vi "Dashboard Main.vi"() -> ()   [LabVIEW 2023]
uses:
  Support/Utility/FP_Size VI to Decoration Simple.vi/TypeDefs_Utility/Cluster_FP Set.ctl
  Support/Utility/FP_Size VI to Decoration Simple.vi/TypeDefs_Utility/ENUM RB_Pos_Quadrant Position.ctl
  <vilib>/event_ctls.llb/eventvkey.ctl
  <vilib>/Rock Robotics/Network Tables/NT Read Numeric Array.vi
  <vilib>/Rock Robotics/WPI/Dashboard/WPI_DashboardLogging Global.vi
panel:
  in  "Camera Settings Right":T1={"Frame Rate"=30, "Compression"=30, "Size"=1, "DB Camera Config"=FALSE} {"Frame Rate" scale=1.0..30.0; "Compression" scale=100.0..-1.0; "Size" items=["640x480", "320x240", "160x120"]}
  in  "Camera Name Right":string(combo)="No Camera Selection"
  out "Camera Perf":string
  in  "Camera Settings":T1={"Frame Rate"=30, "Compression"=30, "Size"=1, "DB Camera Config"=FALSE} {"Frame Rate" scale=1.0..30.0; "Compression" scale=100.0..-1.0; "Size" items=["640x480", "320x240", "160x120"]}
  in  "TCP":refnum<k5>
  in  "Rec Mode":enum32{"Stop", "Record", "Playback"}(radio)
  out "Robot IP":string
  out "Image Message":string="Timeout in Camera Communications"
  in  "Dashboard Tab":T2(tab)
  in  "Select Auto":string(combo)="Select Autonomous ..."
  out "NT Connection":bool
  out "MotorChart R":cluster{"Numeric":dbl, "Numeric":dbl}(graph)
  out "MotorChart L":cluster{"Numeric":dbl, "Numeric":dbl}(graph)
  out "MotorSliders R":cluster{"MotorSlide1":dbl, "MotorSlide2":dbl} {"MotorSlide2" scale=-1.0..1.0 scale format="%#_2e"; "MotorSlide1" scale=-1.0..1.0 scale format="%#_2e"}
  out "MotorSliders L":cluster{"MotorSlide1":dbl, "MotorSlide2":dbl} {"MotorSlide2" scale=-1.0..1.0 scale format="%#_2e"; "MotorSlide1" scale=-1.0..1.0 scale format="%#_2e"}
  out "Gyro":dbl(knob) scale=0.0..360.0
  out "JS1 Z":dbl(slide) scale=-1.0..1.0 scale format="%#_2e"
  out "JS1 Graph":cluster{"X":dbl, "Y":dbl}[](graph)
  out "JS1 Buttons":T3
  out "JS2 Z":dbl(slide) scale=-1.0..1.0 scale format="%#_2e"
  out "JS2 Graph":cluster{"X":dbl, "Y":dbl}[](graph)
  out "JS2 Buttons":T3
  out "Mode":T4(ring)=enum."Auto Disabled"
  out "Right Camera Perf":cluster{"Bandwidth (Mbps)":dbl, "FPS":dbl}
  out "Camera Image Right":T5(plugin-control)
  in  "DB/String 9":string
  in  "DB/String 8":string
  in  "DB/String 7":string
  in  "DB/String 6":string
  in  "DB/String 5":string
  in  "DB/String 4":string
  in  "DB/String 3":string
  in  "DB/String 2":string
  in  "DB/String 1":string
  in  "DB/String 0":string
  in  "DB/Slider 0":dbl(slide) scale=0.0..5.0
  in  "DB/Slider 1":dbl(slide) scale=0.0..5.0
  in  "DB/Slider 2":dbl(slide) scale=0.0..5.0
  in  "DB/Slider 3":dbl(slide) scale=0.0..5.0
  out "DB/LED 3":bool
  out "DB/LED 2":bool
  out "DB/LED 1":bool
  out "DB/LED 0":bool
  in  "DB/Button 3":bool
  in  "DB/Button 2":bool
  in  "DB/Button 1":bool
  in  "DB/Button 0":bool caption="New Name"
  in  "Test Slider":dbl(slide) scale=0.0..100.0 scale format="%#_3g"
  in  "On/Off":bool caption="Solenoid"
  in  "Test Name":u16(ring) items=["Select the test to run..."]
  in  "Test Tree":string(tree)
  in  "Motor":cluster{"Value":dbl, "Enable":bool} {"Value" scale=-1.0..1.0 scale format="%#_3g"}
  out "Progress":T6 {"Test Progress" scale=0.0..100.0}
  in  "Rev/Fwd":cluster{"Forward":bool, "Reverse":bool}
  in  "Test Ring":u16(ring) items=["Monochrome", "Color"]
  in  "CheckList":i32(listbox)
  out "Tree":string(tree)
  out "Camera Image":T5(plugin-control)
  out "Background":bool
  in  "Camera Name":string(combo)="No Camera Selection"
  # "HW"
  # "HW"
  # "Joysticks"
  # "Drive Motors"
  # "Front"
  # "Right"
  # "Left"
  # "Back"
  # "This tab is a great place for autonomous settings and robot-specific values.\nPlace controls and indicators inside this tab and match name to\nDashboard Variables on robot. You can also delete this comment."
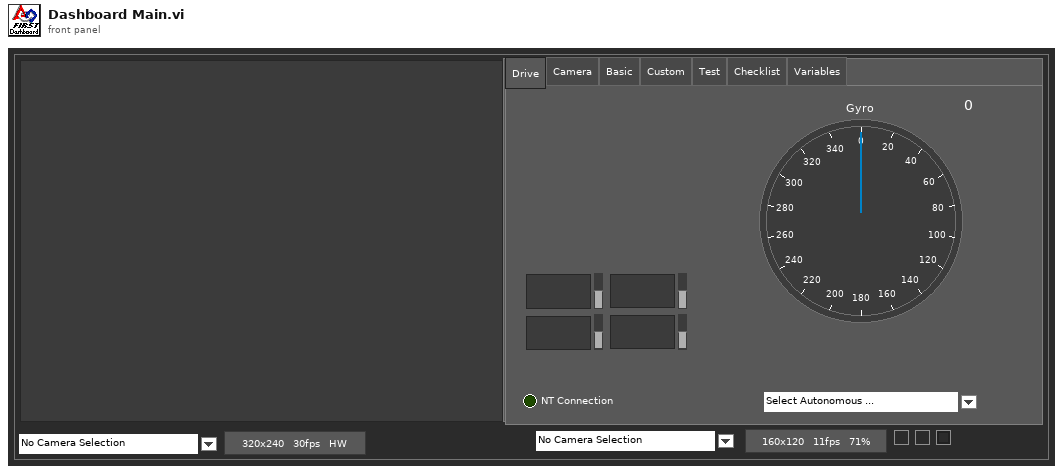
[diagram p1: front panel]
types:
  T1 = cluster{"Frame Rate":i32, "Compression":i32, "Size":u16, "DB Camera Config":bool}
  T2 = enum32{"Drive", "Camera", "Basic", "Custom", "Test", "Checklist", "Variables"}
  T3 = cluster{bool, bool, bool, bool, bool, bool, bool, bool, bool, bool, bool, bool}
  T4 = enum8{"Tele-Op Disabled", "Tele-Op Enabled", "Auto Disabled", "Auto Enabled", "Test Disabled", "Test Enabled", "Disconnected", "No Code", "E-Stop"}
  T5 = typedef "IMAQ Image.ctl" = refnum<image>
  T6 = cluster{"Test Progress":u8, "Test Progress Text":string}
  T7 = typedef "Cluster_FP Set.ctl" = cluster{"Menu Bar":bool, "Position":T8, "Decoration index":i32, "border(px)":i32, "Monitor #":i32}
  T8 = typedef "ENUM RB_Pos_Quadrant Position.ctl" = enum32{"LFT-TOP", "MID-TOP", "RGT-TOP", "LFT-CTR", "MID-CTR", "RGT-CTR", "LFT-BOT", "MID-BOT", "RGT-BOT"}
  T9 = cluster{"Save Path":path, "Interval (s)":dbl, "Keep":i32}
  T10 = enum32{"Drive", "Camera", "Basic", "Custom", "Test", "Commands", "Checklist", "Variables"}
  T11 = typedef "Image Type" = u32
  T12 = cluster{"Error Strings":string, "Disable Counts":cluster{u16, u16}, "Rail Faults":cluster{u16, u16, u16}, "Robot IP":string, "DB Mode":u8, "Event Info":cluster{"Name":string, "Type":u8, "Number":u16, "Replay":u8}}
  T13 = cluster{"Storage":cluster{"Disk Free":u64, "RAM Block":u32, "RAM free":u32}, "CPU Utilization":cluster{"CPU % ISR":sgl, "CPU % Time Crit":sgl, "CPU % Timed Str":sgl, "CPU % High":sgl, "CPU % Above":sgl, "CPU % Normal":sgl, "CPU % Low":sgl}, "CAN":cluster{"% Bus Utilization":sgl, "Bus Off Cnt":u32, "TX_FIFO Full Cnt":u32, "Receive Error Cnt":u8, "Transmit Error Cnt":u8}, "HID":cluster{"HID Outputs":u32, "Rumble Low":u16, "Rumble High":u16}[]}
  T14 = cluster{"Status bits":cluster{"Test Mode":bool, "Autonomous":bool, "Enabled":bool, "Code Start":bool, "Brownout":bool, "Reserved 2":bool, "Reserved 3":bool, "E-Stop":bool}, "Code Trace":cluster{"Disabled":bool, "TeleOp":bool, "Auto":bool, "Test":bool}, "Controller Type":enum16{"unknown", "cRIO", "roboRio"}, "Code?":enum16{"unknown", "noCode", "code"}, "Battery V":dbl}
  T15 = cluster{"Control Bits":cluster{"TestMode":bool, "Autonomous":bool, "Enabled":bool, "FMS Present":bool, bool, bool, bool, "E-Stop":bool}, "Team Station ":u8, "Countdown":sgl, "Joystick Values":cluster{"Axes":dbl[], "Buttons":bool[], "POVs":i16[]}[]}
  T16 = cluster{"Axes":dbl[], "Buttons":bool[], "POVs":i16[]}[]
  T17 = cluster{"Axes":dbl[], "Buttons":bool[], "POVs":i16[]}
  T18 = cluster{"Buttons[0]":bool, "Buttons[1]":bool, "Buttons[2]":bool, "Buttons[3]":bool, "Buttons[4]":bool, "Buttons[5]":bool, "Buttons[6]":bool, "Buttons[7]":bool, "Buttons[8]":bool, "Buttons[9]":bool, "Buttons[10]":bool, "Buttons[11]":bool}
  T19 = cluster{"Global Rectangle":i32[], "Contours":cluster{"Contour Type":u32, "ROI Type":u32, "Points":i32[]}[]}
  T20 = cluster{"Camera Name":string, string, "Saved DB Images Info":cluster{"Save Path":path, "Interval (s)":dbl, "Keep":i32}}
  T21 = cluster{"Camera Name Right":string, string, "Saved DB Images Info":cluster{"Save Path":path, "Interval (s)":dbl, "Keep":i32}}
  T22 = cluster{"Operation":enum16{"Update", "Clear"}, "Color Box":u32}[]
  T23 = typedef "eventvkey.ctl" = enum16{"ASCII", "Enter", "Return", "Shift", "Ctrl", "Alt", "Cmd", "Opt", "Caps", "NumLock", "Clear", "Break", "Up", "Down", "Left", "Right", "Insert", "Delete", "Home", "End", "PageUp", "PageDown", "Escape", "Help", "Pause", "ScrollLock", "F1", "F2", "F3", "F4", "F5", "F6", "F7", "F8", "F9", "F10", "F11", "F12", "F13", "F14", "F15", "F16", "F17", "F18", "F19", "F20", "F21", "F22", "F23", "F24", "Play", "VolumeUp", "VolumeDown", "Mute", "Two Byte Char"}
  T24 = cluster{"Image Size":bool, "Image Type":bool, "Pixel Value":bool, "ROI Information":bool, "Zoom Factor":bool}
  T25 = cluster{"Operation":enum16{"Update", "Clear"}, "Color Box":u32}
  T26 = cluster{"Shift":bool, "Ctrl":bool, "Alt":bool, "Cmd":bool, "Opt":bool}
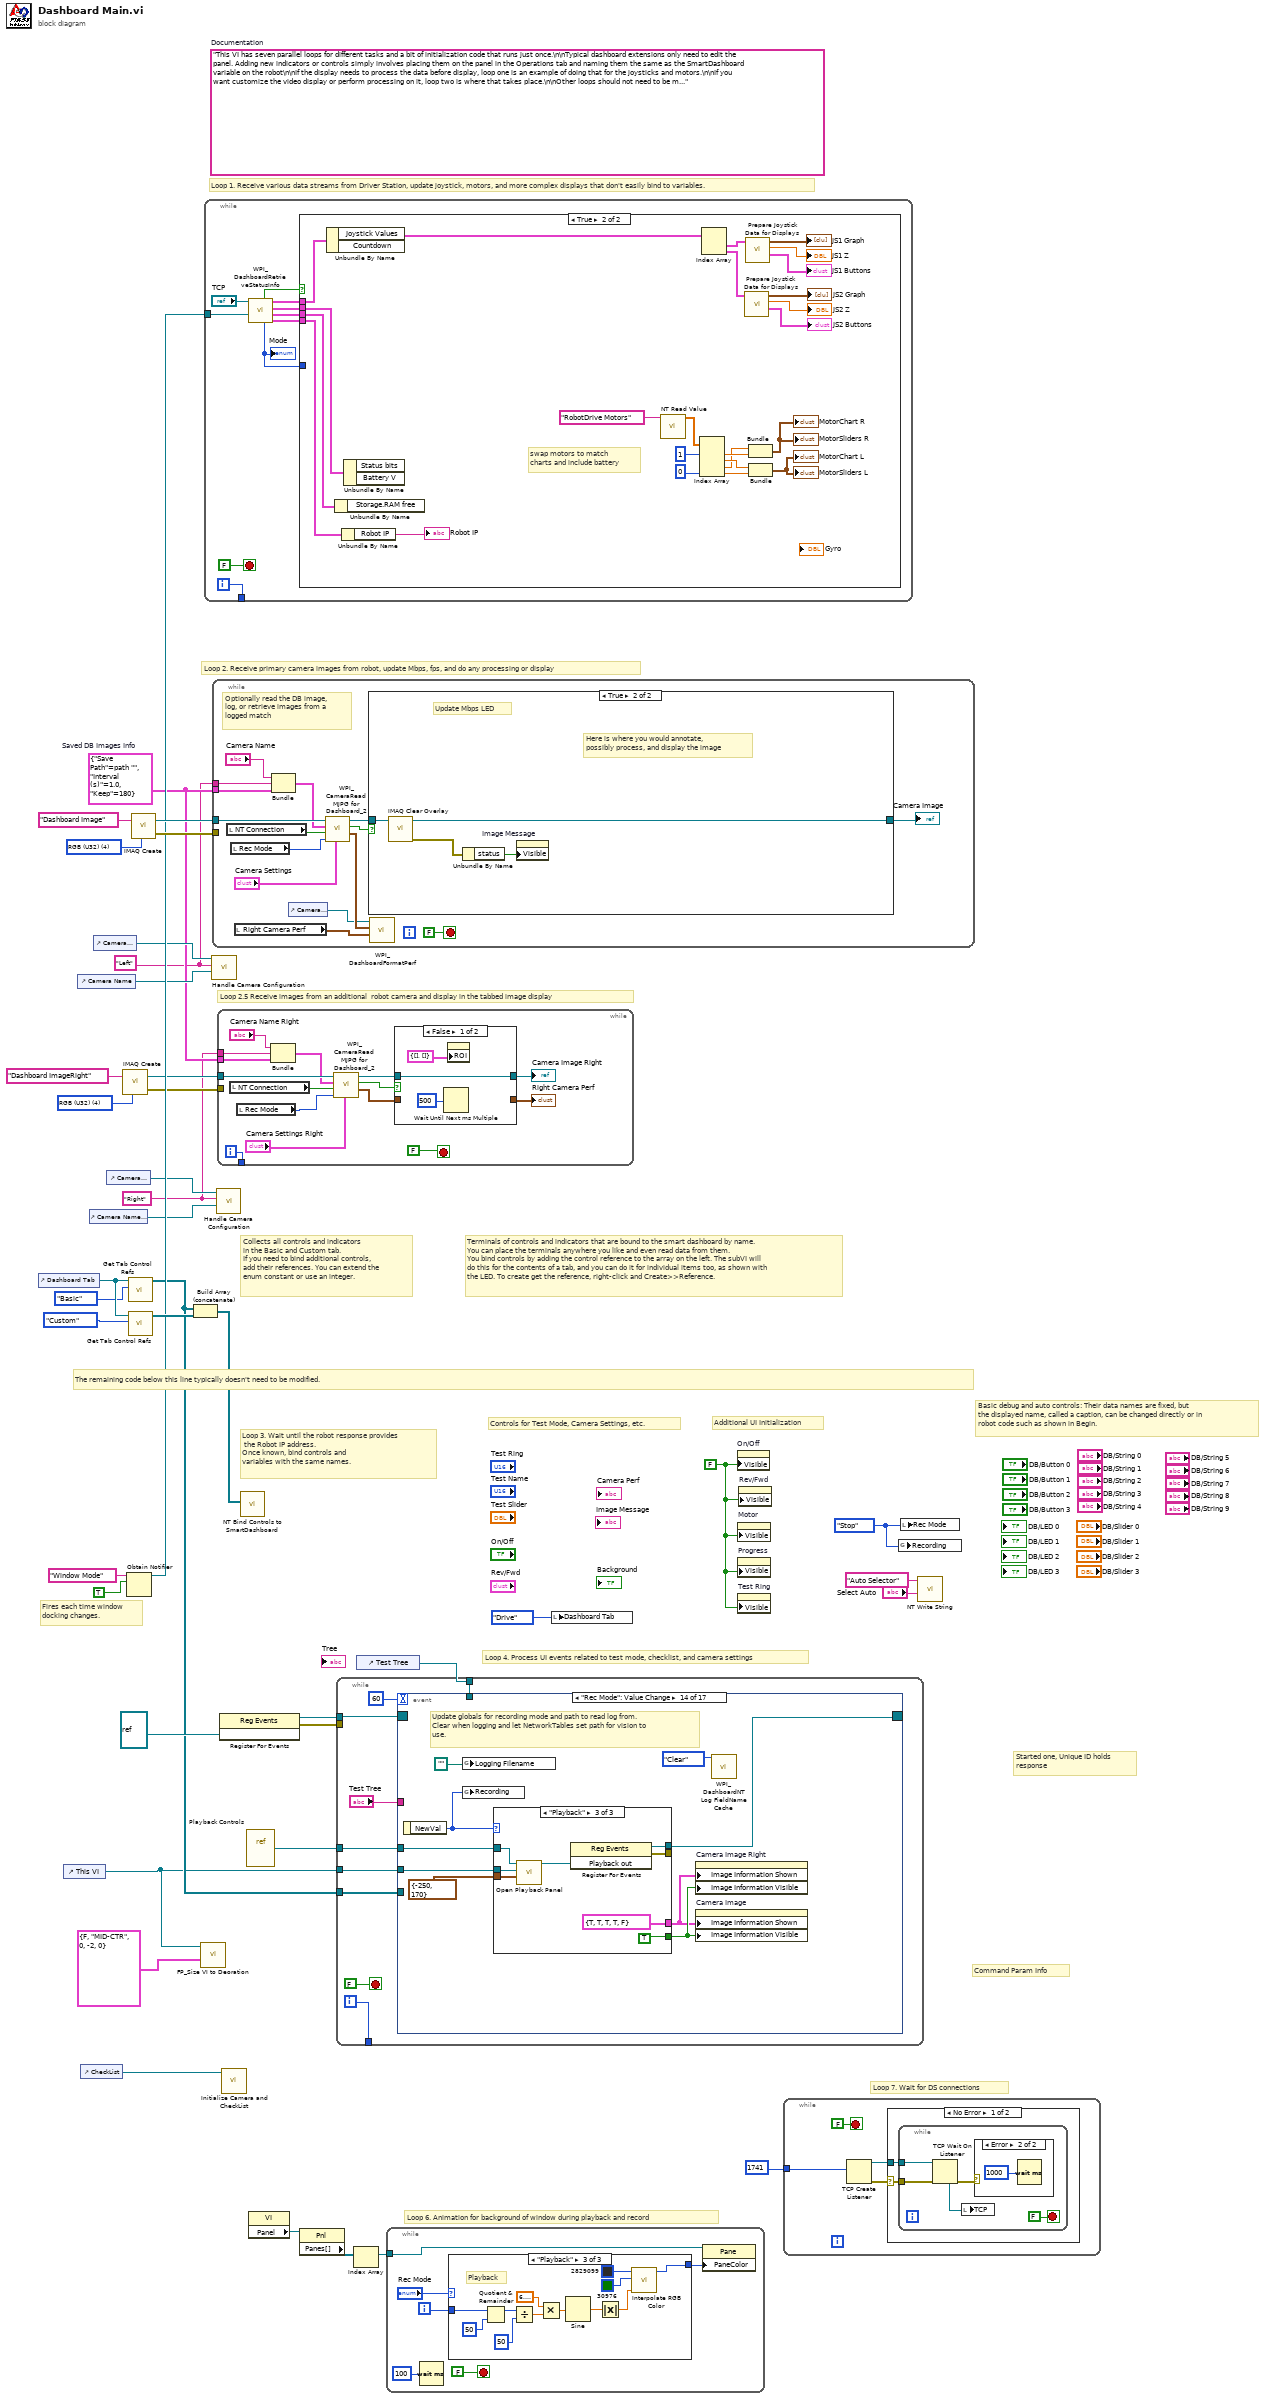
[diagram p0: block diagram]
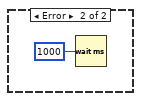
[diagram p4: hidden frame]
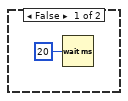
[diagram p5: hidden frame]
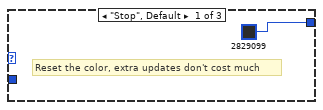
[diagram p6: hidden frame]
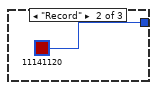
[diagram p7: hidden frame]
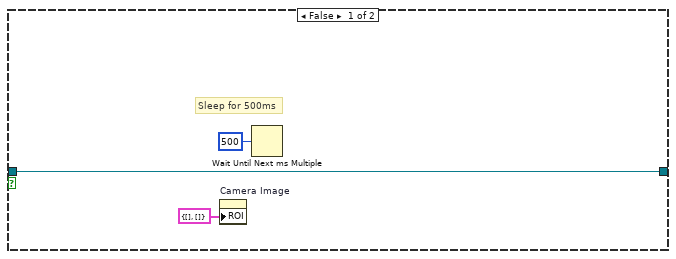
[diagram p8: hidden frame]
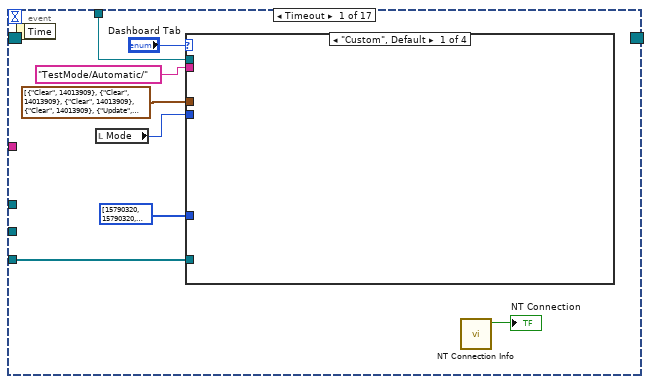
[diagram p9: hidden frame]
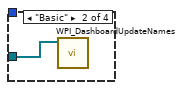
[diagram p10: hidden frame]
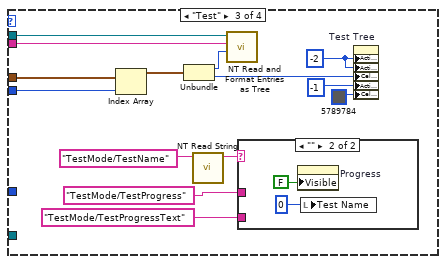
[diagram p11: hidden frame]
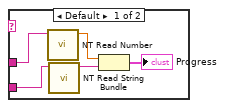
[diagram p12: hidden frame]
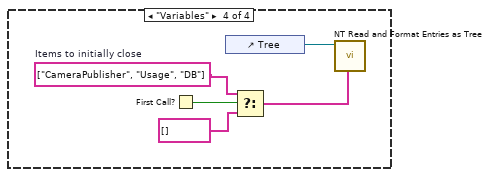
[diagram p13: hidden frame]
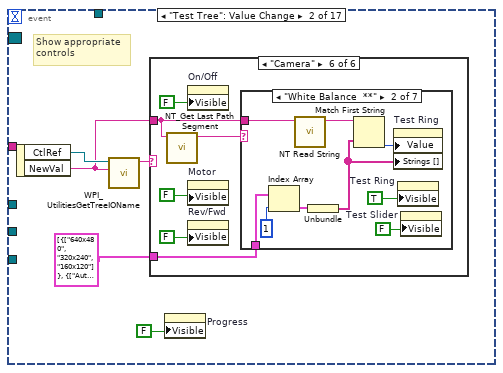
[diagram p14: hidden frame]
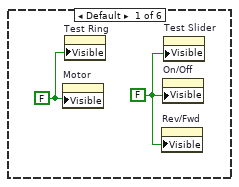
[diagram p15: hidden frame]
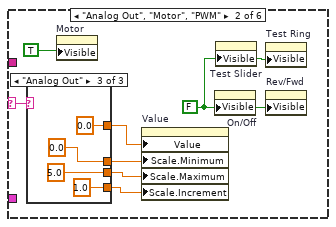
[diagram p16: hidden frame]
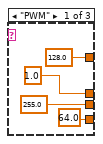
[diagram p17: hidden frame]
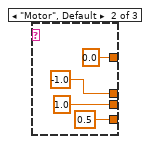
[diagram p18: hidden frame]
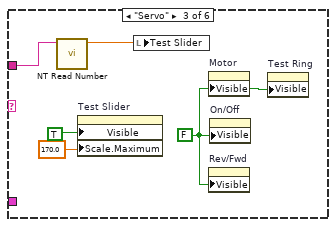
[diagram p19: hidden frame]
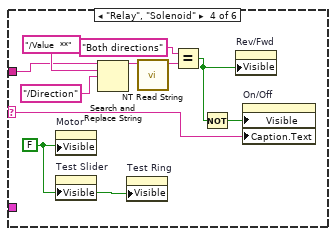
[diagram p20: hidden frame]
diagram:
  w5 = T9 {"Save Path"=path "", "Interval (s)"=1.0, "Keep"=180}  # Saved DB Images Info
  w4 = "Right"
  w3 = "Left"
  w12 = T11 4 items=["Grayscale (U8)", "Grayscale (I16)", "Grayscale (SGL)", "Complex (CSG)", "RGB (U32)", "HSL (U32)", "RGB (U64)"] ("Image Type")
  w27 = enum32{"Stop", "Record", "Playback"}."Stop" ("Rec Mode")
  w22 = FALSE ("Visible")
  (unwired) "This VI has seven parallel loops for different tasks and a bit of initialization code that runs just once.\n\nTypical dashboard extensions only need to edit the panel. Adding new indicators or controls simply involves placing them on the panel in the Operations tab and naming them the same as the SmartDashboard variable on the robot\n\nIf the display needs to process the data before display, loop one is an example of doing that for the joysticks and motors.\n\nIf you want customize the video display or perform processing on it, loop two is where that takes place.\n\nOther loops should not need to be modified. They are pretty standard, and document the task they perform."  # Documentation
  w41 = T11 4 items=["Grayscale (U8)", "Grayscale (I16)", "Grayscale (SGL)", "Complex (CSG)", "RGB (U32)", "HSL (U32)", "RGB (U64)"] ("Image Type")
  # "Loop 2.5 Receive images from an additional  robot camera and display in the tabbed image display"
  # "Command Param Info"
  # "Started one, Unique ID holds\nresponse"
  # "Loop 7. Wait for DS connections"
  # "Basic debug and auto controls: Their data names are fixed, but\nthe displayed name, called a caption, can be changed directly or in\nrobot code such as shown in Begin."
  # "Controls for Test Mode, Camera Settings, etc."
  # "Additional UI Initialization"
  # "Loop 6. Animation for background of window during playback and record"
  # "Fires each time window\ndocking changes."
  # "Collects all controls and indicators\nin the Basic and Custom tab.\nIf you need to bind additional controls,\nadd their references. You can extend the\nenum constant or use an integer."
  # "The remaining code below this line typically doesn't need to be modified."
  # "Loop 4. Process UI events related to test mode, checklist, and camera settings"
  # "Terminals of controls and indicators that are bound to the smart dashboard by name.\nYou can place the terminals anywhere you like and even read data from them.\nYou bind controls by adding the control reference to the array on the left. The subVI will\ndo this for the contents of a tab, and you can do it for individual items too, as shown with\nthe LED. To create get the reference, right-click and Create>>Reference."
  # "Loop 3. Wait until the robot response provides\n the Robot IP address.\nOnce known, bind controls and\nvariables with the same names."
  # "Loop 1. Receive various data streams from Driver Station, update joystick, motors, and more complex displays that don't easily bind to variables."
  # "Loop 2. Receive primary camera images from robot, update Mbps, fps, and do any processing or display"
  n1 = control-ref of="Dashboard Tab"() -> (w26:refnum<vi>)
  n2 = control-ref of="This VI"() -> (w2:refnum<vi>)
  n3 = control-ref of="Camera Name"() -> (w17:refnum<vi>)
  n4 = control-ref of="CheckList"() -> (w23:refnum<vi>)
  n5 = control-ref of="Camera Name Right"() -> (w8:refnum<vi>)
  n6 = control-ref of="Camera Settings"() -> (w18:refnum<vi>)
  n7 = control-ref of="Camera Settings Right"() -> (w9:refnum<vi>)
  n8 = call "IMAQ Create"("Image Name"="Dashboard ImageRight", "Image Type"=w12) -> ("New Image"=w11:T5, "error out"=w10:errorcluster)  [unwired: 2 in, 1 out]
  n9 = Obtain Notifier(name (unnamed)="Window Mode", notification data type=TRUE) -> (notifier out=w21:refnum<notifier>)  [unwired: 2 in, 2 out]
  n10 = call <vilib>:"Get Tab Control Refs.vi"("Page Index"=T10."Basic" ("Dashboard Tab"), "TabControl in"=w26) -> ("ControlsOnPage"=w16:refnum<vi>[])  [unwired: 9 in]
  n11 = call <vilib>:"Get Tab Control Refs.vi"("Page Index"=T10."Custom" ("Dashboard Tab"), "TabControl in"=w26) -> ("ControlsOnPage"=w25:refnum<vi>[])  [unwired: 9 in]
  n12 = call "IMAQ Create"("Image Name"="Dashboard Image", "Image Type"=w41) -> ("New Image"=w39:T5, "error out"=w38:errorcluster)  [unwired: 2 in, 1 out]
  n13 = Build Array (concatenate)(w16, w25) -> (w24:refnum<vi>[])
  n14 = call "FP_Size VI to Deoration.vi"("FPSet"=T7 {"Menu Bar"=FALSE, "Position"=enum."MID-CTR", "Decoration index"=0, "border(px)"=-2, "Monitor #"=0}, "VI Ref"=w2) -> ()  [unwired: 8 in, 2 out]
  n15 = while {
    tunnel: [w50] -> _
    tunnel: w21 -> [w42]
    i -> [w50]
    stop <- FALSE stop-if-true
    n16 = call <vilib>:"WPI_DashboardRetrieveStatusInfo.vi"("Window Mode Notifier"=w42, "TCP Cnx"="TCP") -> ("Power and Errors"=w45:T12, "Robot Metrics"=w48:T13, "Status Info"=w49:T14, "Control Info"=w46:T15, "Robot Mode"=w44:T4, "Process?"=w47:bool)  [unwired: 4 in]
    "Mode" <- w44
    n17 = case shown="True" w47 {
      tunnel: w49 -> [_ w76]
      tunnel: w48 -> [_ w75]
      tunnel: w46 -> [_ w74]
      tunnel: w45 -> [_ w73]
      tunnel: w44 -> [_ _]
      frame False {
        n18 = Wait (ms)(milliseconds to wait=u32 20) -> ()  [unwired: 1 out]
      }
      frame True {
        # "swap motors to match\ncharts and include battery"
        n19 = Unbundle By Name(w74) -> ("Joystick Values"=w64:T16)  [unwired: 1 out]
        n20 = Unbundle By Name(w75) -> ()  [unwired: 1 out]
        n21 = Unbundle By Name(w73) -> ("Robot IP"=→"Robot IP":string)
        n22 = Unbundle By Name(w76) -> ()  [unwired: 2 out]
        n23 = call-poly <vilib>:"NT Read Value.vi"("name"="RobotDrive Motors" ("Name")) -> ("value"=w54:dbl[])  [unwired: 8 in, 2 out]
        n24 = Index Array(array=w54, index #1=1, index #4=0) -> (element #1=w68:dbl, element #2=w69:dbl, element #3=w67:dbl, element #4=w72:dbl)  [unwired: 2 in]
        n25 = Index Array(array=w64) -> (element #1=w63:T17, element #2=w59:T17)  [unwired: 2 in]
        n26 = call "Prepare Joystick Data for Displays.vi"("Joystick Values"=w59) -> ("Buttons"=→"JS2 Buttons":T18, "Z Axis"=→"JS2 Z":dbl, "Cartesian Data"=→"JS2 Graph":cluster{"X axis":dbl, "X axis":dbl}[])  [unwired: 8 in]
        n27 = call "Prepare Joystick Data for Displays.vi"("Joystick Values"=w63) -> ("Buttons"=→"JS1 Buttons":T18, "Z Axis"=→"JS1 Z":dbl, "Cartesian Data"=→"JS1 Graph":cluster{"X axis":dbl, "X axis":dbl}[])  [unwired: 8 in]
        n28 = Bundle("Numeric"=w67, "Numeric"=w68) -> (→"MotorChart R" →"MotorSliders R":cluster{"Numeric":dbl, "Numeric":dbl})  [unwired: 1 in]
        n29 = Bundle("Numeric"=w69, "Numeric"=w72) -> (→"MotorChart L" →"MotorSliders L":cluster{"Numeric":dbl, "Numeric":dbl})  [unwired: 1 in]
      }
    }
  }
  n30 = call "Handle Camera Configuration.vi"("CameraNameRef"=w17, "Display Name"=w3, "ClusterRef"=w18) -> ()  [unwired: 9 in]
  n31 = while {
    tunnel: w39 -> [w90]
    tunnel: w38 -> [_]
    tunnel: w5 -> [w83]
    tunnel: w3 -> [w80]
    stop <- FALSE stop-if-true
    # "Optionally read the DB image,\nlog, or retrieve images from a\nlogged match"
    n32 = local read "NT Connection"() -> (w84:bool)
    n33 = local read "Rec Mode"() -> (w87:enum32{"Stop", "Record", "Playback"})
    n34 = local read "Right Camera Perf"() -> (w78:cluster{"Bandwidth (Mbps)":dbl, "FPS":dbl})
    n35 = Bundle("Camera Name"="Camera Name", w80, "Saved DB Images Info"=w83) -> (w82:T20)  [unwired: 1 in]
    n36 = control-ref of="Camera Perf"() -> (w77:refnum<vi>)
    n37 = call <vilib>:"WPI_CameraRead MJPG for Dashboard_2.vi"("Camera Settings"="Camera Settings", "Rec Mode"=w87, "NT Connection"=w84, "Capture Info"=w82, "Image in"=w90) -> ("perf info"=w79:cluster{"Bandwidth (Mbps)":dbl, "fps":dbl}, "Active"=w88:bool, "Image\\ out"=w89:T5)  [unwired: 4 in]
    n38 = case shown="True" w88 {
      tunnel: w89 -> [w93 w96]
      tunnel: [w93 w95] -> w85
      frame False {
        # "Sleep for 500ms"
        n39 = property on="Camera Image" class="ImageControl"("ROI"=T19 {"Global Rectangle"=[], "Contours"=[]}) -> ()  [unwired: 2 in, 2 out]
        n40 = Wait Until Next ms Multiple(millisecond multiple=u32 500) -> ()  [unwired: 1 out]
      }
      frame True {
        # "Here is where you would annotate,\npossibly process, and display the image"
        # "Update Mbps LED"
        n41 = call "IMAQ Clear Overlay"("Image"=w96) -> ("error out"=w97:errorcluster, "Image Out"=w95:T5)  [unwired: 2 in, 7 out]
        n42 = Unbundle By Name(w97) -> ("status"=w98:bool)
        n43 = property on="Image Message" class="Str"("Visible"=w98) -> ()  [unwired: 2 in, 2 out]
      }
    }
    "Camera Image" <- w85
    n44 = call <vilib>:"WPI_DashboardFormatPerf.vi"("Right Camera Perf"=w78, "Performance"=w79, "String in"=w77) -> ()  [unwired: 9 in]
  }
  n45 = call "Handle Camera Configuration.vi"("CameraNameRef"=w8, "Display Name"=w4, "ClusterRef"=w9) -> ()  [unwired: 9 in]
  n46 = while {
    tunnel: w11 -> [w113]
    tunnel: w10 -> [_]
    tunnel: [w108] -> _
    tunnel: w5 -> [w104]
    tunnel: w4 -> [w101]
    i -> [w108]
    stop <- FALSE stop-if-true
    n47 = local read "NT Connection"() -> (w105:bool)
    n48 = local read "Rec Mode"() -> (w112:enum32{"Stop", "Record", "Playback"})
    n49 = Bundle("Camera Name Right"="Camera Name Right", w101, "Saved DB Images Info"=w104) -> (w103:T21)  [unwired: 1 in]
    n50 = call <vilib>:"WPI_CameraRead MJPG for Dashboard_2.vi"("Camera Settings"="Camera Settings Right", "Rec Mode"=w112, "NT Connection"=w105, "Capture Info"=w103, "Image in"=w113) -> ("perf info"=w99:cluster{"Bandwidth (Mbps)":dbl, "fps":dbl}, "Active"=w107:bool, "Image\\ out"=w110:T5)  [unwired: 4 in]
    n51 = case shown="False" w107 {
      tunnel: w110 -> [w115 w118]
      tunnel: [w115 w118] -> w106
      tunnel: [_ w117] -> w100
      tunnel: w99 -> [_ w117]
      frame False {
        n52 = Wait Until Next ms Multiple(millisecond multiple=u32 500) -> ()  [unwired: 1 out]
        n53 = property on="Camera Image Right" class="ImageControl"("ROI"=T19 {"Global Rectangle"=[], "Contours"=[]}) -> ()  [unwired: 2 in, 2 out]
      }
      frame True {
      }
    }
    "Camera Image Right" <- w106
    "Right Camera Perf" <- w100
  }
  n54 = register-events(refnum<vi> refnum) -> (reference out=w30:refnum<event-registration>, error out=w29:errorcluster)  [unwired: 2 in]
  n55 = call "Initialize Camera and CheckList.vi"("ListBox in"=w23) -> ()  [unwired: 11 in]
  n56 = call <vilib>:"NT Bind Controls to SmartDashboard.vi"("Bound Control Refs"=w24) -> ()  [unwired: 11 in]
  n57 = vi-ref "Playback Controls.vi"() -> (w31:refnum<vi>)
  n58 = property class="VI"() -> ("Panel"=w33:refnum<vi>)  [unwired: 2 in, 2 out]
  n59 = property class="Pnl"(reference=w33) -> ("Panes[]"=w34:refnum<vi>[])  [unwired: 1 in, 2 out]
  n60 = Index Array(array=w34) -> (element=w32:refnum<vi>)  [unwired: 1 in]
  n61 = control-ref of="Test Tree"() -> (w35:refnum<vi>)
  n62 = while {
    tunnel: [w124] -> _
    tunnel: w35 -> [w123]
    tunnel: w31 -> [w122]
    tunnel: w30 -> [w121]
    tunnel: w29 -> [_]
    tunnel: w2 -> [w120]
    tunnel: w16 -> [w119]
    i -> [w124]
    stop <- FALSE stop-if-true
    n63 = event shown="[13] \"Rec Mode\": Value Change" {
      selector: w121 -> [_ _ _ _ _ _ _ _ _ _ _ _ _ _ _ _ _]
      dyn-events: [_ _ _ _ _ _ _ _ _ _ _ _ _ w329 _ _ _] -> _
      timeout: u32 60 ("milliseconds to wait") -> [_ _ _ _ _ _ _ _ _ _ _ _ _ _ _ _ _]
      tunnel: w123 -> [w134 _ _ _ _ _ _ _ _ _ _ _ _ _ _ _ _]
      tunnel: "Test Tree" -> [_ _ _ _ _ _ _ _ w302 w309 w310 w313 w320 _ _ _ _]
      tunnel: w122 -> [_ _ _ _ _ _ _ _ _ _ _ _ _ w331 _ w346 _]
      tunnel: w120 -> [_ _ _ _ _ _ _ _ _ _ _ _ _ w327 _ _ _]
      tunnel: w119 -> [w129 _ _ _ _ _ _ _ _ _ _ _ _ _ _ _ _]
      event Timeout {
        n64 = event-data() -> ()  [unwired: 1 in, 1 out]
        n65 = local read "Mode"() -> (w132:T4)
        n66 = case shown="\"Custom\", Default" "Dashboard Tab" {
          tunnel: w134 -> [_ _ w150 _]
          tunnel: "TestMode/Automatic/" ("Name Pattern") -> [_ _ w149 _]
          tunnel: T22 [{"Operation"=enum."Clear", "Color Box"=14013909}, {"Operation"=enum."Clear", "Color Box"=14013909}, {"Operation"=enum."Clear", "Color Box"=14013909}, {"Operation"=enum."Clear", "Color Box"=14013909}, {"Operation"=enum."Update", "Color Box"=14013909}, {"Operation"=enum."Update", "Color Box"=16777215}, {"Operation"=enum."Clear", "Color Box"=14013909}, {"Operation"=enum."Clear", "Color Box"=14013909}, {"Operation"=enum."Clear", "Color Box"=14013909}] -> [_ _ w142 _]
          tunnel: w132 -> [_ _ w141 _]
          tunnel: u32[] [15790320, 15790320, 15790320, 15790320, 16777215, 16777215, 15790320, 15790320, 15790320] -> [_ _ _ _]
          tunnel: w129 -> [_ w136 _ _]
          frame "Custom", Default {
          }
          frame "Basic" {
            n67 = call <vilib>:"WPI_DashboardUpdateNames.vi"("Controls on Tab"=w136) -> ()  [unwired: 11 in]
          }
          frame "Test" {
            w148 = -2 ("Active Item:Row Number")
            n68 = Index Array(array=w142, index=w141) -> (element=w143:T25)
            n69 = Unbundle(w143) -> ("Operation"=w144:enum16{"Update", "Clear"}, "Color Box"=w145:u32)
            n70 = call <vilib>:"NT Read String.vi"("name"="TestMode/TestName" ("Name")) -> ("value"=w139:string)  [unwired: 8 in, 2 out]
            n71 = call <vilib>:"NT Read and Format Entries as Tree.vi"("Operation"=w144, "Name Pattern"=w149, "Tree Refnum"=w150) -> ()  [unwired: 7 in, 2 out]
            n72 = case shown="\"\"" w139 {
              tunnel: "TestMode/TestProgress" ("Name") -> [w152 _]
              tunnel: "TestMode/TestProgressText" ("Name") -> [w151 _]
              frame Default {
                n73 = call <vilib>:"NT Read Number.vi"("name"=w152) -> ("value"=w153:dbl)  [unwired: 8 in, 2 out]
                n74 = call <vilib>:"NT Read String.vi"("name"=w151) -> ("value"=w154:string)  [unwired: 8 in, 2 out]
                n75 = Bundle("value"=w153, "value"=w154) -> (→"Progress":cluster{"value":dbl, "value":string})  [unwired: 1 in]
              }
              frame "" {
                n76 = property on="Progress" class="Clust (strict)"("Visible"=FALSE) -> ()  [unwired: 2 in, 2 out]
                n77 = local write "Test Name"(u16 0) -> ()
              }
            }
            n78 = property on="Test Tree" class="Tree (strict)"("Active Item Row Number"=w148, "ActiveColNum"=w148, "CellBG"=w145, "Active Item Row Number"=-1 ("Active Item:Row Number"), "CellBG"=u32 5789784 ("Color Box")) -> ()  [unwired: 2 in, 2 out]
          }
          frame "Variables" {
            w160 = string[] ["CameraPublisher", "Usage", "DB"]  # Items to initially close
            n79 = First Call?() -> (First Call?: T/F=w161:bool)
            n80 = control-ref of="Tree"() -> (w162:refnum<vi>)
            n81 = Select(t=w160, s=w161, f=string[] []) -> (s? t:f=w158:string[])
            n82 = call <vilib>:"NT Read and Format Entries as Tree.vi"("Tags to  Close"=w158, "Tree Refnum"=w162) -> ()  [unwired: 8 in, 2 out]
          }
        }
        n83 = call <vilib>:"NT Connection Info.vi"() -> ("Connected"=→"NT Connection":bool)  [unwired: 11 in]
      }
      event "Test Tree": Value Change {
        # "Show appropriate\ncontrols"
        n84 = event-data() -> ("CtlRef"=w166:refnum<vi>, "NewVal"=w164:string)  [unwired: 1 in]
        n85 = call <vilib>:"WPI_UtilitiesGetTreeIOName.vi"("NewVal"=w164, "TreeControl in"=w166) -> ("I/O Name"=w167:string)  [unwired: 9 in]
        n86 = case shown="\"Camera\"" w167 {
          selector: w167 -> [_ w174 _ w196 w205 _]
          tunnel: w164 -> [_ _ w193 w195 _ w212]
          tunnel: cluster{string[]}[] [{["640x480", "320x240", "160x120"]}, {["Auto", "Fixed indoor", "Fixed outdoor 1", "Fixed outdoor 2", "Fixed fluorescent 1", "Fixed fluorescent 2", "Hold current"]}, {["Auto", "Flicker-free 50 Hz", "Flicker-free 60 Hz", "Hold current"]}, {["None", "Prioritize frame rate", "Prioritize image quality"]}, {["Monochrome", "Color"]}] -> [_ _ _ _ _ w211]
          frame Default {
            w169 = FALSE ("Visible")
            w168 = FALSE ("Visible")
            n87 = property on="Motor" class="Clust (strict)"("Visible"=w168) -> ()  [unwired: 2 in, 2 out]
            n88 = property on="Test Ring" class="Ring (strict)"("Visible"=w168) -> ()  [unwired: 2 in, 2 out]
            n89 = property on="Rev/Fwd" class="Clust (strict)"("Visible"=w169) -> ()  [unwired: 2 in, 2 out]
            n90 = property on="On/Off" class="Bool (strict)"("Visible"=w169) -> ()  [unwired: 2 in, 2 out]
            n91 = property on="Test Slider" class="Slide (strict)"("Visible"=w169) -> ()  [unwired: 2 in, 2 out]
          }
          frame "Analog Out", "Motor", "PWM" {
            w175 = FALSE ("Visible")
            n92 = case shown="\"Analog Out\"" w174 {
              tunnel: [1.0 ("Value") -1.0 ("Value") 0.0 ("Value")] -> w173
              tunnel: [255.0 ("Value") 1.0 ("Value") 5.0 ("Value")] -> w172
              tunnel: [128.0 ("Value") 0.0 ("Value") 0.0 ("Value")] -> w171
              tunnel: [64.0 ("Value") 0.5 ("Value") 1.0 ("Value")] -> w170
              frame "PWM" {
              }
              frame "Motor", Default {
              }
              frame "Analog Out" {
              }
            }
            n93 = property on="Motor" class="Clust (strict)"("Visible"=TRUE) -> ()  [unwired: 2 in, 2 out]
            n94 = property on="Value" class="Slide (strict)"("Value"=w171, "Scale.Minimum"=w173, "Scale.Maximum"=w172, "Scale.Increment"=w170) -> ()  [unwired: 2 in, 2 out]
            n95 = property on="On/Off" class="Bool (strict)"("Visible"=w175) -> ()  [unwired: 2 in, 2 out]
            n96 = property on="Test Slider" class="Slide (strict)"("Visible"=w175) -> ()  [unwired: 2 in, 2 out]
            n97 = property on="Test Ring" class="Ring (strict)"("Visible"=w175) -> ()  [unwired: 2 in, 2 out]
            n98 = property on="Rev/Fwd" class="Clust (strict)"("Visible"=w175) -> ()  [unwired: 2 in, 2 out]
          }
          frame "Servo" {
            w191 = FALSE ("Visible")
            n99 = call <vilib>:"NT Read Number.vi"("name"=w193) -> ("value"=w192:dbl)  [unwired: 8 in, 2 out]
            n100 = property on="Test Slider" class="Slide (strict)"("Visible"=TRUE, "Scale.Maximum"=170.0 ("Scale.Range:Maximum")) -> ()  [unwired: 2 in, 2 out]
            n101 = local write "Test Slider"(w192) -> ()
            n102 = property on="Motor" class="Clust (strict)"("Visible"=w191) -> ()  [unwired: 2 in, 2 out]
            n103 = property on="Rev/Fwd" class="Clust (strict)"("Visible"=w191) -> ()  [unwired: 2 in, 2 out]
            n104 = property on="On/Off" class="Bool (strict)"("Visible"=w191) -> ()  [unwired: 2 in, 2 out]
            n105 = property on="Test Ring" class="Ring (strict)"("Visible"=w191) -> ()  [unwired: 2 in, 2 out]
          }
          frame "Relay", "Solenoid" {
            w194 = FALSE ("Visible")
            n106 = property on="Motor" class="Clust (strict)"("Visible"=w194) -> ()  [unwired: 2 in, 2 out]
            n107 = property on="Test Slider" class="Slide (strict)"("Visible"=w194) -> ()  [unwired: 2 in, 2 out]
            n108 = Search and Replace String(input string=w195, search string="/Value  **", replace string="/Direction") -> (result string=w201:string)  [unwired: 5 in, 3 out]
            n109 = property on="Test Ring" class="Ring (strict)"("Visible"=w194) -> ()  [unwired: 2 in, 2 out]
            n110 = call <vilib>:"NT Read String.vi"("name"=w201) -> ("value"=w199:string)  [unwired: 8 in, 2 out]
            n111 = Equal?(x="Both directions", y=w199) -> (x = y?=w197:bool)
            n112 = Not(x=w197) -> (.not. x?=w198:bool)
            n113 = property on="Rev/Fwd" class="Clust (strict)"("Visible"=w197) -> ()  [unwired: 2 in, 2 out]
            n114 = property on="On/Off" class="Bool (strict)"("Visible"=w198, "Caption.Text"=w196) -> ()  [unwired: 2 in, 2 out]
          }
          frame "Compressor", "Digital Out" {
            w204 = FALSE ("Visible")
            # "Get direction and finish"
            n115 = property on="Motor" class="Clust (strict)"("Visible"=w204) -> ()  [unwired: 2 in, 2 out]
            n116 = property on="Test Slider" class="Slide (strict)"("Visible"=w204) -> ()  [unwired: 2 in, 2 out]
            n117 = property on="Test Ring" class="Ring (strict)"("Visible"=w204) -> ()  [unwired: 2 in, 2 out]
            n118 = property on="On/Off" class="Bool (strict)"("Visible"=TRUE, "Caption.Text"=w205) -> ()  [unwired: 2 in, 2 out]
            n119 = property on="Rev/Fwd" class="Clust (strict)"("Visible"=FALSE) -> ()  [unwired: 2 in, 2 out]
          }
          frame "Camera" {
            n120 = call <vilib>:"NT_Get Last Path Segment.vi"("String in"=w212) -> ("String out"=w213:string)  [unwired: 10 in]
            n121 = property on="On/Off" class="Bool (strict)"("Visible"=FALSE) -> ()  [unwired: 2 in, 2 out]
            n122 = property on="Motor" class="Clust (strict)"("Visible"=FALSE) -> ()  [unwired: 2 in, 2 out]
            n123 = property on="Rev/Fwd" class="Clust (strict)"("Visible"=FALSE) -> ()  [unwired: 2 in, 2 out]
            n124 = case shown="\"White Balance  **\"" w213 {
              tunnel: w212 -> [w219 w228 w237 w246 w255 _ w261]
              tunnel: w211 -> [w217 w225 w234 w243 w252 _ _]
              frame "Size  **" {
                n125 = Index Array(array=w217) -> (element=w216:cluster{string[]})  [unwired: 1 in]
                n126 = call <vilib>:"NT Read String.vi"("name"=w219) -> ("value"=w218:string)  [unwired: 8 in, 2 out]
                n127 = Unbundle(w216) -> (w214:string[])
                n128 = Match First String(2:w214, 3:w218) -> (0:w215:i32)  [unwired: 1 out]
                n129 = property on="Test Ring" class="Ring (strict)"("Value"=w215, "Strings []"=w214) -> ()  [unwired: 2 in, 2 out]
                n130 = property on="Test Ring" class="Ring (strict)"("Visible"=TRUE) -> ()  [unwired: 2 in, 2 out]
                n131 = property on="Test Slider" class="Slide (strict)"("Visible"=FALSE) -> ()  [unwired: 2 in, 2 out]
              }
              frame "White Balance  **" {
                n132 = Index Array(array=w225, index=1) -> (element=w226:cluster{string[]})
                n133 = call <vilib>:"NT Read String.vi"("name"=w228) -> ("value"=w227:string)  [unwired: 8 in, 2 out]
                n134 = Unbundle(w226) -> (w223:string[])
                n135 = Match First String(2:w223, 3:w227) -> (0:w222:i32)  [unwired: 1 out]
                n136 = property on="Test Ring" class="Ring (strict)"("Value"=w222, "Strings []"=w223) -> ()  [unwired: 2 in, 2 out]
                n137 = property on="Test Ring" class="Ring (strict)"("Visible"=TRUE) -> ()  [unwired: 2 in, 2 out]
                n138 = property on="Test Slider" class="Slide (strict)"("Visible"=FALSE) -> ()  [unwired: 2 in, 2 out]
              }
              frame "Exposure  **" {
                n139 = Index Array(array=w234, index=2) -> (element=w235:cluster{string[]})
                n140 = call <vilib>:"NT Read String.vi"("name"=w237) -> ("value"=w236:string)  [unwired: 8 in, 2 out]
                n141 = Unbundle(w235) -> (w231:string[])
                n142 = Match First String(2:w231, 3:w236) -> (0:w232:i32)  [unwired: 1 out]
                n143 = property on="Test Ring" class="Ring (strict)"("Value"=w232, "Strings []"=w231) -> ()  [unwired: 2 in, 2 out]
                n144 = property on="Test Ring" class="Ring (strict)"("Visible"=TRUE) -> ()  [unwired: 2 in, 2 out]
                n145 = property on="Test Slider" class="Slide (strict)"("Visible"=FALSE) -> ()  [unwired: 2 in, 2 out]
              }
              frame "Exposure Priority  **" {
                n146 = Index Array(array=w243, index=3) -> (element=w244:cluster{string[]})
                n147 = call <vilib>:"NT Read String.vi"("name"=w246) -> ("value"=w245:string)  [unwired: 8 in, 2 out]
                n148 = Unbundle(w244) -> (w240:string[])
                n149 = Match First String(2:w240, 3:w245) -> (0:w241:i32)  [unwired: 1 out]
                n150 = property on="Test Ring" class="Ring (strict)"("Value"=w241, "Strings []"=w240) -> ()  [unwired: 2 in, 2 out]
                n151 = property on="Test Ring" class="Ring (strict)"("Visible"=TRUE) -> ()  [unwired: 2 in, 2 out]
                n152 = property on="Test Slider" class="Slide (strict)"("Visible"=FALSE) -> ()  [unwired: 2 in, 2 out]
              }
              frame "Color Enable  **" {
                n153 = Index Array(array=w252, index=4) -> (element=w253:cluster{string[]})
                n154 = call <vilib>:"NT Read String.vi"("name"=w255) -> ("value"=w254:string)  [unwired: 8 in, 2 out]
                n155 = Unbundle(w253) -> (w249:string[])
                n156 = Match First String(2:w249, 3:w254) -> (0:w250:i32)  [unwired: 1 out]
                n157 = property on="Test Ring" class="Ring (strict)"("Value"=w250, "Strings []"=w249) -> ()  [unwired: 2 in, 2 out]
                n158 = property on="Test Ring" class="Ring (strict)"("Visible"=TRUE) -> ()  [unwired: 2 in, 2 out]
                n159 = property on="Test Slider" class="Slide (strict)"("Visible"=FALSE) -> ()  [unwired: 2 in, 2 out]
              }
              frame Default {
                n160 = property on="Test Ring" class="Ring (strict)"("Visible"=FALSE) -> ()  [unwired: 2 in, 2 out]
                n161 = property on="Test Slider" class="Slide (strict)"("Visible"=FALSE) -> ()  [unwired: 2 in, 2 out]
              }
              frame "Brightness  **", "Color Level  **", "Compression  **", "FPS  **", "Sharpness  **" {
                n162 = call <vilib>:"NT Read Number.vi"("name"=w261) -> ("value"=w260:dbl)  [unwired: 8 in, 2 out]
                n163 = local write "Test Slider"(w260) -> ()
                n164 = property on="Test Ring" class="Ring (strict)"("Visible"=FALSE) -> ()  [unwired: 2 in, 2 out]
                n165 = property on="Test Slider" class="Slide (strict)"("Visible"=TRUE, "Scale.Maximum"=100.0 ("Scale.Range:Maximum")) -> ()  [unwired: 2 in, 2 out]
              }
            }
          }
        }
        n166 = property on="Progress" class="Clust (strict)"("Visible"=FALSE) -> ()  [unwired: 2 in, 2 out]
      }
      event "Test Name": Mouse Enter {
        # "Populate the ring with the list of tests"
        n167 = event-data() -> ()  [unwired: 1 in, 1 out]
        n168 = call <vilib>:"NT Read String Array.vi"("name"="TestMode/TestList" ("Name")) -> ("value"=w268:string[])  [unwired: 8 in, 2 out]
        n169 = Build Array (concatenate)("Select the test to run...", w268) -> (w267:string[])
        n170 = property on="Test Name" class="Ring (strict)"("Strings []"=w267) -> ()  [unwired: 2 in, 2 out]
      }
      event "Test Name": Value Change {
        w269 = FALSE ("Visible")
        # "Tell the robot the test name to run"
        n171 = event-data() -> ("NewVal"=w273:u16)  [unwired: 1 in]
        n172 = property on="Test Name" class="Ring (strict)"() -> ("Strings []"=w274:string[])  [unwired: 2 in, 2 out]
        n173 = local write "Progress"(T6 {"Test Progress"=0, "Test Progress Text"=""} ("Progress")) -> ()
        n174 = Index Array(array=w274, index=w273) -> (element=w272:string)
        n175 = call <vilib>:"NT Write String.vi"("value"=w272, "name"="TestMode/TestName" ("Name")) -> ()  [unwired: 9 in, 1 out]
        n176 = property on="Progress" class="Clust (strict)"("Visible"=TRUE) -> ()  [unwired: 2 in, 2 out]
        n177 = property on="Motor" class="Clust (strict)"("Visible"=w269) -> ()  [unwired: 2 in, 2 out]
        n178 = property on="Test Slider" class="Slide (strict)"("Visible"=w269) -> ()  [unwired: 2 in, 2 out]
        n179 = property on="On/Off" class="Bool (strict)"("Visible"=w269) -> ()  [unwired: 2 in, 2 out]
        n180 = property on="Rev/Fwd" class="Clust (strict)"("Visible"=w269) -> ()  [unwired: 2 in, 2 out]
        n181 = property on="Test Ring" class="Ring (strict)"("Visible"=w269) -> ()  [unwired: 2 in, 2 out]
      }
      event "Select Auto": Mouse Enter {
        # "Populate the combo box with the list of autonomous options"
        n182 = event-data() -> ()  [unwired: 1 in, 1 out]
        n183 = call <vilib>:"NT Read String Array.vi"("name"="Auto List" ("Name")) -> ("value"=w276:string[])  [unwired: 8 in, 2 out]
        n184 = property on="Select Auto" class="CmbBox"("Strings[]"=w276) -> ()  [unwired: 2 in, 2 out]
      }
      event "Select Auto": Value Change {
        # "User modified the Auto Selection. Write to NT variable so robot knows."
        n185 = event-data() -> ("NewVal"=w278:string)  [unwired: 1 in]
        n186 = call <vilib>:"NT Write String.vi"("value"=w278, "name"="Auto Selector" ("Name")) -> ()  [unwired: 9 in, 1 out]
      }
      event "CheckList": Double Click {
        # "Shift clears all"
        # "Update symbols on the listbox"
        n187 = event-data() -> ("PlatMods.Shift"=w280:bool, "Row"=w282:i32)  [unwired: 1 in]
        n188 = case shown="True" w280 {
          tunnel: w282 -> [w286 _]
          tunnel: 1 -> [w285 _]
          frame False {
            n189 = property on="CheckList" class="LstBox (strict)"() -> ("Item Symbols"=w284:i32[])  [unwired: 2 in, 2 out]
            n190 = Replace Array Subset(array=w284, new element=w285, index=w286) -> (w283:i32[])
            n191 = property on="CheckList" class="LstBox (strict)"("Item Symbols"=w283) -> ()  [unwired: 2 in, 2 out]
          }
          frame True {
            w287 = 0 ("Top Row")
            n192 = property on="CheckList" class="LstBox (strict)"() -> ("Number of Rows"=w289:u32)  [unwired: 2 in, 2 out]
            n193 = Initialize Array(0, w289) -> (w288:i32[])
            n194 = property on="CheckList" class="LstBox (strict)"("Top Row"=w287, "Value"=w287, "Item Symbols"=w288) -> ()  [unwired: 2 in, 2 out]
          }
        }
      }
      event "CheckList": Key Down {
        # "Update symbols on the listbox\nLeft and right keys check and uncheck"
        n195 = event-data() -> ("VKey"=w292:T23)  [unwired: 1 in]
        n196 = case shown="\"Left\", \"Right\"" w292 {
          selector: w292 -> [w297 _]
          tunnel: eventvkey."Left" ("VKey") -> [w295 _]
          frame "Left", "Right" {
            n197 = Equal?(x=w295, y=w297) -> (x = y?=w296:bool)
            n198 = Select(t=0, s=w296, f=1) -> (s? t:f=w298:i32)
            n199 = property on="CheckList" class="LstBox (strict)"() -> ("Item Symbols"=w301:i32[])  [unwired: 2 in, 2 out]
            n200 = Replace Array Subset(array=w301, new element=w298, index="CheckList") -> (w300:i32[])
            n201 = property on="CheckList" class="LstBox (strict)"("Item Symbols"=w300) -> ()  [unwired: 2 in, 2 out]
          }
          frame Default {
          }
        }
      }
      event "Motor.Enable": Value Change {
        # "When the test mode otor enable helper is set, update that\ntree row item's value"
        n202 = event-data() -> ("NewVal"=w306:bool)  [unwired: 1 in]
        n203 = Unbundle("Motor") -> ("Value"=w305:dbl)  [unwired: 1 out]
        n204 = Select(t=w305, s=w306, f=0.0) -> (s? t:f=w303:dbl)
        n205 = call <vilib>:"NT Write Number.vi"("value"=w303, "name"=w302) -> ()  [unwired: 9 in, 1 out]
      }
      event "Test Slider": Value Change {
        # "When the test mode slider helper is set, update that\ntree row item's value"
        n206 = event-data() -> ("NewVal"=w308:dbl)  [unwired: 1 in]
        n207 = call <vilib>:"NT Write Number.vi"("value"=w308, "name"=w309) -> ()  [unwired: 9 in, 1 out]
      }
      event "On/Off": Value Change {
        # "When the test mode on/off helper value is set, update that\ntree row item's value"
        n208 = event-data() -> ("NewVal"=w312:bool)  [unwired: 1 in]
        n209 = Boolean To (0,1)(Boolean=w312) -> (0, 1=w311:i16)
        n210 = call <vilib>:"NT Write Number.vi"("value"=w311, "name"=w310) -> ()  [unwired: 9 in, 1 out]
      }
      event "Rev/Fwd": Value Change {
        # "When the test mode helper value for relays is set, update that\ntree row item's value"
        n211 = event-data() -> ("NewVal.Forward"=w319:bool, "NewVal.Reverse"=w318:bool)  [unwired: 1 in]
        n212 = Boolean To (0,1)(Boolean=w319) -> (0, 1=w315:i16)
        n213 = Boolean To (0,1)(Boolean=w318) -> (0, 1=w317:i16)
        n214 = Negate(x=w317) -> (-x=w316:i16)
        n215 = Add(x=w315, y=w316) -> (x+y=w314:i16)
        n216 = call <vilib>:"NT Write Number.vi"("value"=w314, "name"=w313) -> ()  [unwired: 9 in, 1 out]
      }
      event "Test Ring": Value Change {
        # "When a test mode helper value is selected from the ring,\nset the tree item's variable to the string value"
        n217 = event-data() -> ("NewVal"=w322:u16)  [unwired: 1 in]
        n218 = property on="Test Ring" class="Ring (strict)"() -> ("Strings []"=w323:string[])  [unwired: 2 in, 2 out]
        n219 = Index Array(array=w323, index=w322) -> (element=w321:string)
        n220 = call <vilib>:"NT Write String.vi"("value"=w321, "name"=w320) -> ()  [unwired: 9 in, 1 out]
      }
      event "Rec Mode": Value Change {
        # "Update globals for recording mode and path to read log from.\nClear when logging and let NetworkTables set path for vision to\nuse."
        n221 = event-data() -> ("NewVal"=w332:enum32{"Stop", "Record", "Playback"})  [unwired: 1 in]
        n222 = global write "WPI_DashboardLogging Global.vi" "Logging Filename"(path "") -> ()
        n223 = global write "WPI_DashboardLogging Global.vi" "Recording"(w332) -> ()
        n224 = case shown="\"Playback\"" w332 {
          tunnel: w331 -> [_ w334 w342]
          tunnel: [_ _ w341] -> w329
          tunnel: [_ _ w340] -> _
          tunnel: w327 -> [_ _ w338]
          tunnel: cluster{i32, i32} {-250, 170} -> [_ _ w337]
          tunnel: [_ _ T24 {"Image Size"=TRUE, "Image Type"=TRUE, "Pixel Value"=TRUE, "ROI Information"=TRUE, "Zoom Factor"=FALSE} ("Image Information Shown:All Elements")] -> w324
          tunnel: [_ _ TRUE ("Zoom Factor")] -> w325
          frame Default {
          }
          frame "Stop", "Record" {
            # "Place Window too"
            n225 = invoke class="VI" method="FP.Close"(reference=w334) -> (reference out=w333:refnum<vi>)  [unwired: 2 in, 2 out]
            n226 = invoke class="VI" method="Abort VI"(reference=w333) -> ()  [unwired: 2 in, 3 out]
          }
          frame "Playback" {
            n227 = call "Open Playback Panel.vi"("Offset"=w337, "DB VI Ref"=w338, "Playback in"=w342) -> ("Playback out"=w339:refnum<vi>)  [unwired: 8 in]
            n228 = register-events(w339) -> (reference out=w341:refnum<event-registration>, error out=w340:errorcluster)  [unwired: 2 in]
          }
        }
        n229 = property on="Camera Image Right" class="ImageControl"("Image Information Shown"=w324, "Image Information Visible"=w325) -> ()  [unwired: 2 in, 2 out]
        n230 = property on="Camera Image" class="ImageControl"("Image Information Shown"=w324, "Image Information Visible"=w325) -> ()  [unwired: 2 in, 2 out]
        n231 = call <vilib>:"WPI_DashboardNT Log FieldName Cache.vi"("Operation"=enum16{"Lookup/Add", "Index", "Clear"}."Clear") -> ()  [unwired: 8 in, 3 out]
      }
      event Panel Close {
        w343 = enum32{"Stop", "Record", "Playback"}."Stop" ("Rec Mode")
        # "Playback window has been closed, abort"
        n232 = event-data() -> ()  [unwired: 1 in, 4 out]
        n233 = local write "Rec Mode"(w343) -> ()
        n234 = global write "WPI_DashboardLogging Global.vi" "Recording"(w343) -> ()
      }
      event Panel Close {
        # "Abort playback window and ourself"
        n235 = event-data() -> ()  [unwired: 1 in, 4 out]
        n236 = invoke class="VI" method="FP.Close"(reference=w346) -> (reference out=w345:refnum<vi>)  [unwired: 2 in, 2 out]
        n237 = invoke class="VI" method="Abort VI"(reference=w345) -> (error out=w344:errorcluster)  [unwired: 2 in, 2 out]
        n238 = invoke class="VI" method="Abort VI"(error in=w344) -> ()  [unwired: 2 in, 3 out]
      }
      event "Tree": Double Click {
        n239 = event-data() -> ("PlatMods"=w352:T26, "Tag"=w349:string)  [unwired: 1 in]
        n240 = Unbundle(w352) -> ("Shift"=w351:bool)  [unwired: 4 out]
        n241 = String Subset(string=w349, length (rest)=1 ("length (rest)")) -> (substring=w348:string)  [unwired: 1 in]
        n242 = Not(x=w351) -> (.not. x?=w350:bool)
        n243 = case shown="\"/\"" w348 {
          tunnel: w349 -> [_ w354]
          tunnel: w350 -> [_ w353]
          frame Default {
          }
          frame "/" {
            n244 = call <vilib>:"NT Update Persistence.vi"("Persistence"=w353, "Name"=w354) -> ()  [unwired: 9 in, 1 out]
          }
        }
      }
    }
  }
  n245 = while {
    tunnel: w32 -> [w356]
    i -> [w359]
    stop <- FALSE stop-if-true
    n246 = Wait (ms)(milliseconds to wait=u32 100) -> ()  [unwired: 1 out]
    n247 = case shown="\"Playback\"" "Rec Mode" {
      tunnel: w359 -> [_ _ w374]
      tunnel: [u32 2829099 ("Base Color") u32 11141120 ("Target Color") w363] -> w355
      frame "Stop", Default {
        # "Reset the color, extra updates don't cost much"
      }
      frame "Record" {
      }
      frame "Playback" {
        # "Playback"
        n248 = Quotient & Remainder(x=w374, y=u32 50 ("milliseconds to wait")) -> (x-y*floor(x/y)=w370:u32)  [unwired: 1 out]
        n249 = Divide(x=w370, y=u32 50 ("milliseconds to wait")) -> (x/y=w367:dbl)
        n250 = Multiply(x=6.283185307179586, y=w367) -> (x*y=w372:dbl)
        n251 = Sine(x=w372) -> (sin(x)=w371:dbl)
        n252 = Absolute Value(x=w371) -> (abs(x)=w364:dbl)
        n253 = call "Interpolate RGB Color.vi"("Proportion"=w364, "Target Color"=u32 30976, "Base Color"=u32 2829099) -> ("Result Color"=w363:u32)  [unwired: 8 in]
      }
    }
    n254 = property class="Pane"(reference=w356, "PaneColor"=w355) -> ()  [unwired: 1 in, 2 out]
  }
  n255 = local write "Dashboard Tab"(T2."Drive" ("Dashboard Tab")) -> ()
  n256 = property on="On/Off" class="Bool (strict)"("Visible"=w22) -> ()  [unwired: 2 in, 2 out]
  n257 = property on="Motor" class="Clust (strict)"("Visible"=w22) -> ()  [unwired: 2 in, 2 out]
  n258 = property on="Progress" class="Clust (strict)"("Visible"=w22) -> ()  [unwired: 2 in, 2 out]
  n259 = property on="Test Ring" class="Ring (strict)"("Visible"=w22) -> ()  [unwired: 2 in, 2 out]
  n260 = property on="Rev/Fwd" class="Clust (strict)"("Visible"=w22) -> ()  [unwired: 2 in, 2 out]
  n261 = while {
    tunnel: u16 1741 ("timeout ms (25000)") -> [w376]
    stop <- FALSE stop-if-true
    n262 = TCP Create Listener(10:w376) -> (0:w375:errorcluster, 3:w377:refnum<k5>)  [unwired: 4 in, 1 out]
    n263 = case shown="No Error" w375 {
      selector: w375 -> [w379 _]
      tunnel: w377 -> [w380 _]
      frame No Error {
        n264 = while {
          tunnel: w380 -> [w383]
          tunnel: w379 -> [w382]
          stop <- FALSE stop-if-true
          n265 = TCP Wait On Listener(8:w382, 11:w383) -> (0:w384:errorcluster, 4:w385:refnum<k5>)  [unwired: 2 in, 3 out]
          n266 = local write "TCP"(w385) -> ()
          n267 = case shown="Error" w384 {
            frame No Error {
            }
            frame Error {
              n268 = Wait (ms)(milliseconds to wait=u32 1000) -> ()  [unwired: 1 out]
            }
          }
        }
      }
      frame Error {
        n269 = Wait (ms)(milliseconds to wait=u32 1000) -> ()  [unwired: 1 out]
      }
    }
  }
  n270 = global write "WPI_DashboardLogging Global.vi" "Recording"(w27) -> ()
  n271 = local write "Rec Mode"(w27) -> ()
  n272 = call <vilib>:"NT Write String.vi"("value"="Select Auto", "name"="Auto Selector" ("Name")) -> ()  [unwired: 9 in, 1 out]
